vi "Connect to PC Beamage.vi"(8 "error in":errorcluster) -> (0 "error out":errorcluster, 1 "Connected":bool)   [LabVIEW 2009]
uses:
  BeamageNP.dll
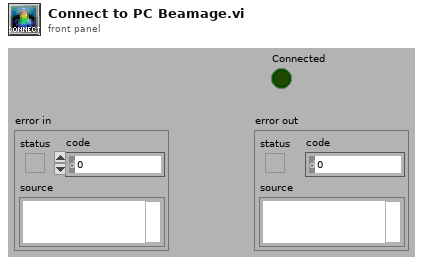
[diagram p1: front panel]
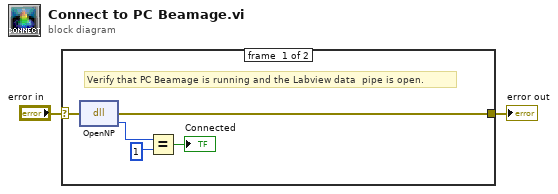
[diagram p0: block diagram]
diagram:
  n1 = case shown="No Error" "error in" {
    selector: "error in" -> [w4 w8]
    tunnel: [w3 w8] -> w1
    frame #0 {
      # "Verify that PC Beamage is running and the Labview data  pipe is open."
      n2 = dll-call lib="S:/LabView Files/Beamage 3.0/BeamageNP.dll" fn="OpenNP"(error in=w4) -> (error out=w3:errorcluster, "return type"=w7:i32)  [unwired: 2 in, 1 out]
      n3 = Equal?(x=w7, y=1) -> (x = y?=→"Connected":bool)
    }
    frame #1 {
    }
  }
  "error out" <- w1
